vi "Fetch Multi Eval Meas Power Dynamics Results.vi"(8 "error in (no error)":errorcluster, 9 "Result Type (Current)":i32(ring) items=["Current"=0, "Average"=1, "Standard Deviation"=3, "Maximum"=4, "Minimum"=5], 10 "Instance (1)":T2=1, 11 "VISA resource name":refnum<visa-resource-name>) -> (0 "error out":errorcluster, 1 "Power Dynamics Results":T1 {"Off Power After" format="%^.3e"; "On Power Peak" format="%^.3e"; "On Power RMS" format="%^.3e"; "Off Power Before" format="%^.3e"}, 2 "Reliability":i32, 3 "VISA resource name out":refnum<visa-resource-name>, 5 "Out Of Tolerance":i32)   [LabVIEW 2020, in "Rohde&Schwarz CMWXP NR FR1 Measurement.lvlib"]
doc: "Return the current, average, minimum, maximum and standard deviation single value results of the power dynamics measurement.\n\nAttributes:\nRSCMWXPNRFR1M_ATTR_FETCH_MULTI_MEAS_EVAL_POWER_DYNAMICS_CURRENT_RESULTS\nRSCMWXPNRFR1M_ATTR_FETCH_MULTI_MEAS_EVAL_POWER_DYNAMICS_AVERAGE_RESULTS\nRSCMWXPNRFR1M_ATTR_FETCH_MULTI_MEAS_EVAL_POWER_DYNAMICS_STANDARD_DEVIATION_RESULTS\nRSCMWXPNRFR1M_ATTR_FETCH_MULTI_MEAS_EVAL_POWER_DYNAMICS_MAXIMUM_RESULTS\nRSCMWXPNRFR1M_ATTR_FETCH_MULTI_MEAS_EVAL_POWER_DYNAMICS_MINIMUM_RESULTS\n\nRemote-control commands:\nFETCh:NRSub:MEAS<i>:MEValuation:PDYNamics:CURRent?\nFETCh:NRSub:MEAS<i>:MEValuation:PDYNamics:AVERage?\nFETCh:NRSub:MEAS<i>:MEValuation:PDYNamics:SDEViation?\nFETCh:NRSub:MEAS<i>:MEValuation:PDYNamics:MAXimum?\nFETCh:NRSub:MEAS<i>:MEValuation:PDYNamics:MINimum?"
uses:
  <instrlib>/Rohde&Schwarz CMWXP NR FR1 Measurement/Rohde&Schwarz CMWXP NR FR1 Measurement.lvlib
  <instrlib>/Rohde&Schwarz CMWXP NR FR1 Measurement/Private/_Instance.ctl
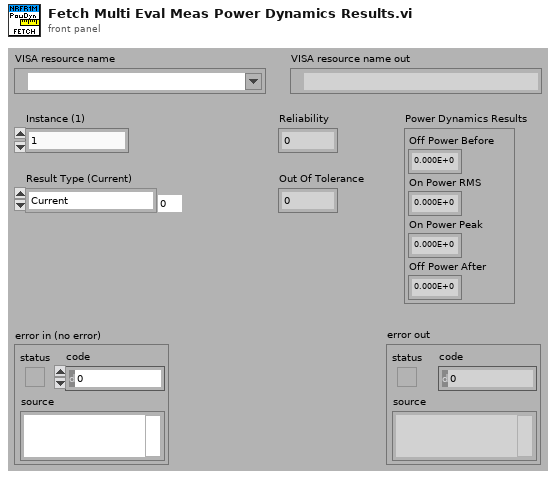
[diagram p1: front panel]
types:
  T1 = cluster{"Off Power Before":dbl, "On Power RMS":dbl, "On Power Peak":dbl, "Off Power After":dbl}
  T2 = typedef "Rohde&Schwarz CMWXP NR FR1 Measurement.lvlib/_Instance.ctl" = i32
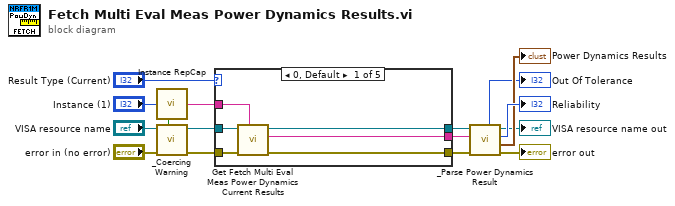
[diagram p0: block diagram]
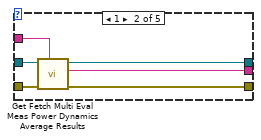
[diagram p2: hidden frame]
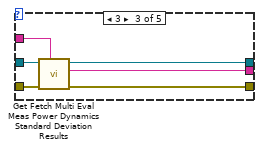
[diagram p3: hidden frame]
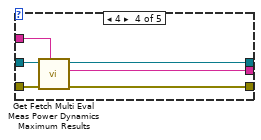
[diagram p4: hidden frame]
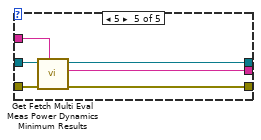
[diagram p5: hidden frame]
diagram:
  n1 = call <instrlib>:"Instance RepCap.vi"("Instance In"="Instance (1)") -> ("In Range?"=w13:bool, "RepCap Identifier Out"=w12:string)  [unwired: 1 in]
  n2 = call <instrlib>:"_Coercing Warning.vi"("In Range?"=w13, "error in (no error)"="error in (no error)", "VISA resource name"="VISA resource name") -> ("error out"=w10:errorcluster, "VISA resource name out"=w11:refnum<visa-resource-name>)  [unwired: 7 in]
  n3 = case shown="0, Default" "Result Type (Current)" {
    tunnel: w12 -> [w22 w28 w34 w40 w46]
    tunnel: w11 -> [w21 w27 w33 w39 w45]
    tunnel: w10 -> [w20 w26 w32 w38 w44]
    tunnel: [w19 w25 w31 w37 w43] -> w6
    tunnel: [w18 w24 w30 w36 w42] -> w7
    tunnel: [w17 w23 w29 w35 w41] -> w8
    frame 0, Default {
      n4 = call "Get Fetch Multi Eval Meas Power Dynamics Current Results"("Repeated Capabilities"=w22, "error in (no error)"=w20, "instrument handle"=w21) -> ("error out"=w17:errorcluster, "Fetch Multi Eval Meas Power Dynamics Current Results"=w18:string, "instrument handle out"=w19:refnum<visa-resource-name>)  [unwired: 6 in]
    }
    frame 1 {
      n5 = call "Get Fetch Multi Eval Meas Power Dynamics Average Results"("Repeated Capabilities"=w28, "error in (no error)"=w26, "instrument handle"=w27) -> ("error out"=w23:errorcluster, "Fetch Multi Eval Meas Power Dynamics Average Results"=w24:string, "instrument handle out"=w25:refnum<visa-resource-name>)  [unwired: 6 in]
    }
    frame 3 {
      n6 = call "Get Fetch Multi Eval Meas Power Dynamics Standard Deviation Results"("Repeated Capabilities"=w34, "error in (no error)"=w32, "instrument handle"=w33) -> ("error out"=w29:errorcluster, "Fetch Multi Eval Meas Power Dynamics Standard Deviation Results"=w30:string, "instrument handle out"=w31:refnum<visa-resource-name>)  [unwired: 6 in]
    }
    frame 4 {
      n7 = call "Get Fetch Multi Eval Meas Power Dynamics Maximum Results"("Repeated Capabilities"=w40, "error in (no error)"=w38, "instrument handle"=w39) -> ("error out"=w35:errorcluster, "Fetch Multi Eval Meas Power Dynamics Maximum Results"=w36:string, "instrument handle out"=w37:refnum<visa-resource-name>)  [unwired: 6 in]
    }
    frame 5 {
      n8 = call "Get Fetch Multi Eval Meas Power Dynamics Minimum Results"("Repeated Capabilities"=w46, "error in (no error)"=w44, "instrument handle"=w45) -> ("error out"=w41:errorcluster, "Fetch Multi Eval Meas Power Dynamics Minimum Results"=w42:string, "instrument handle out"=w43:refnum<visa-resource-name>)  [unwired: 6 in]
    }
  }
  n9 = call <instrlib>:"_Parse Power Dynamics Result.vi"("error in (no error)"=w8, "Input String"=w7, "VISA resource name"=w6) -> ("error out"=→"error out":errorcluster, "Power Dynamics Results"=→"Power Dynamics Results":T1, "Reliability"=→"Reliability":i32, "VISA resource name out"=→"VISA resource name out":refnum<visa-resource-name>, "Out Of Tolerance"=→"Out Of Tolerance":i32)  [unwired: 4 in]
